vi "Module Not Stopped--error.vi"() -> (0 "error out":errorcluster)   [LabVIEW 2015, in "TestStand Manager_DQMH.lvlib"]
doc: "Outputs an error cluster containing a custom error code indicating the Stop Module VI timed out while waiting for the module main VI to stop.\n_____\nBased on Delacor QMH Project Template 2.0.0.62.\n\n<b>Note:</b> This VI was modified by the <b>Validate DQMH Module</b> tool to upgrade it to the DQMH 2.1 approach to stopping a singleton module.\n____\nDelacor QMH Thermal Chamber Examples 4.0.0.21\nCopyright (c) 2018, Delacor"
uses:
  TestStand Manager_DQMH.lvlib
  <vilib>/Utility/error.llb/Error Cluster From Error Code.vi
  <vilib>/ErrorRing/Error Ring.xnode
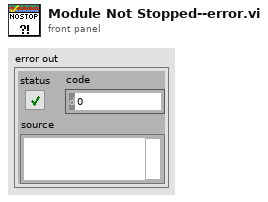
[diagram p1: front panel]
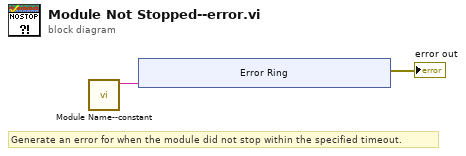
[diagram p0: block diagram]
diagram:
  # "Generate an error for when the module did not stop within the specified timeout."
  n1 = call "Module Name--constant.vi"() -> ("Module Name"=w1:string)  [unwired: 11 in]
  n2 = xnode "Error Ring"("parameter 0"=w1) -> ("error out"=→"error out":errorcluster)
